vi "myRIO_BRig_Host_parse_dataTrial__v3.vi"(0 "input_idxReward":i32, 1 "input_arrayReward":i32[][](array[numeric]), 2 "input_idxWrong":i32, 3 "input_arrayWrong":i32[][](array[numeric]), 4 "input_idxTimeout":i32, 5 "input_arrayTimeout":i32[][](array[numeric]), 6 "input_arrayUnknown":i32[][](array[numeric]), 8 "input_idxUnknown":i32) -> (14 "output_plotData":cluster{i32[], i32[]}[](array[cluster]))   [LabVIEW 2014]
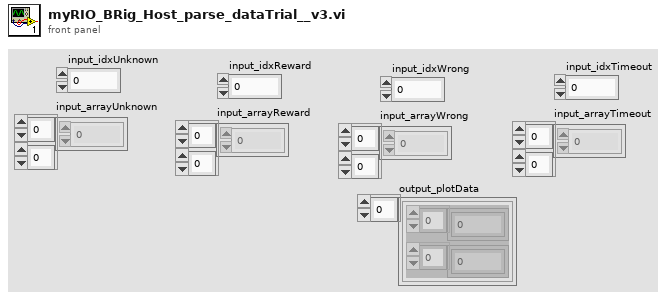
[diagram p1: front panel]
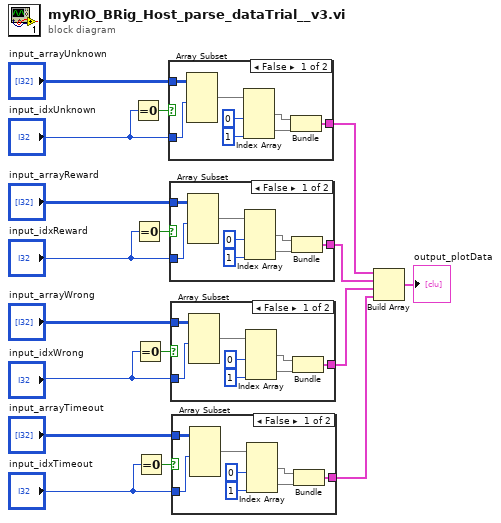
[diagram p0: block diagram]
diagram:
  n1 = Equal To 0?(x="input_idxUnknown") -> (x = 0?=w15:bool)
  n2 = Equal To 0?(x="input_idxReward") -> (x = 0?=w14:bool)
  n3 = Equal To 0?(x="input_idxWrong") -> (x = 0?=w13:bool)
  n4 = Equal To 0?(x="input_idxTimeout") -> (x = 0?=w12:bool)
  n5 = case shown="False" w15 {
    tunnel: "input_arrayUnknown" -> [w25 _]
    tunnel: "input_idxUnknown" -> [w18 _]
    tunnel: [w19 _] -> w3
    frame False {
      n6 = Array Subset(array=w25, length (row)=w18) -> (w24:i32[][])  [unwired: 3 in]
      n7 = Index Array(array=w24, index (col) #1=0 ("disabled index (col)"), index (col) #2=1 ("index (col)")) -> (element #1=w21:i32[], element #2=w20:i32[])  [unwired: 2 in]
      n8 = Bundle(w21, w20) -> (w19:cluster{i32[], i32[]})  [unwired: 1 in]
    }
    frame True {
    }
  }
  n9 = case shown="False" w14 {
    tunnel: "input_arrayReward" -> [w33 _]
    tunnel: "input_idxReward" -> [w27 _]
    tunnel: [w26 _] -> w5
    frame False {
      n10 = Array Subset(array=w33, length (row)=w27) -> (w32:i32[][])  [unwired: 3 in]
      n11 = Index Array(array=w32, index (col) #1=0 ("disabled index (col)"), index (col) #2=1 ("index (col)")) -> (element #1=w29:i32[], element #2=w28:i32[])  [unwired: 2 in]
      n12 = Bundle(w29, w28) -> (w26:cluster{i32[], i32[]})  [unwired: 1 in]
    }
    frame True {
    }
  }
  n13 = case shown="False" w13 {
    tunnel: "input_arrayWrong" -> [w41 _]
    tunnel: "input_idxWrong" -> [w35 _]
    tunnel: [w34 _] -> w4
    frame False {
      n14 = Array Subset(array=w41, length (row)=w35) -> (w40:i32[][])  [unwired: 3 in]
      n15 = Index Array(array=w40, index (col) #1=0 ("disabled index (col)"), index (col) #2=1 ("index (col)")) -> (element #1=w37:i32[], element #2=w36:i32[])  [unwired: 2 in]
      n16 = Bundle(w37, w36) -> (w34:cluster{i32[], i32[]})  [unwired: 1 in]
    }
    frame True {
    }
  }
  n17 = case shown="False" w12 {
    tunnel: "input_arrayTimeout" -> [w49 _]
    tunnel: "input_idxTimeout" -> [w43 _]
    tunnel: [w42 _] -> w2
    frame False {
      n18 = Array Subset(array=w49, length (row)=w43) -> (w48:i32[][])  [unwired: 3 in]
      n19 = Index Array(array=w48, index (col) #1=0 ("disabled index (col)"), index (col) #2=1 ("index (col)")) -> (element #1=w45:i32[], element #2=w44:i32[])  [unwired: 2 in]
      n20 = Bundle(w45, w44) -> (w42:cluster{i32[], i32[]})  [unwired: 1 in]
    }
    frame True {
    }
  }
  n21 = Build Array(w3, w5, w4, w2) -> (→"output_plotData":cluster{i32[], i32[]}[])
